vi "HH_ToImageOffline.vi"(0 "Data In":u32[](array[numeric]), 1 "Reset":bool, 2 "Image Array In":i32[][](array[numeric]), 5 "Data Count":i32, 9 "Pixel Time (Laser Pulses)":i32, 11 "Trace Bins":i32=25) -> (3 "Image Array Out":i32[][](array[numeric]), 4 "Histograms":i32[][](array[numeric]), 6 "Total Photon Count":u64[](array[numeric]), 8 "Trigger Times":u64[](array[numeric]), 13 "Total Oveflow Count":u64, 14 "Num Records Total":i64, 15 "Traces":i32[][](array[numeric]))   [LabVIEW 2011]
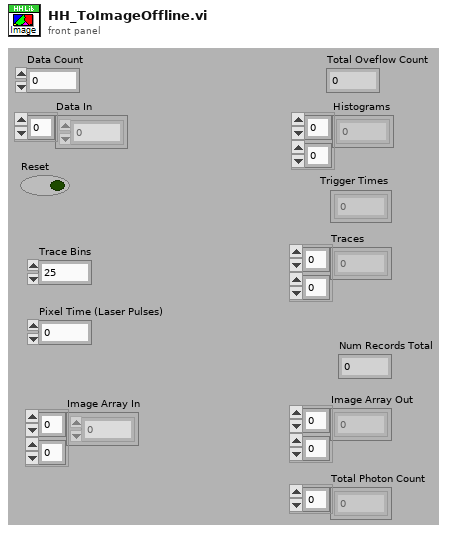
[diagram p1: front panel]
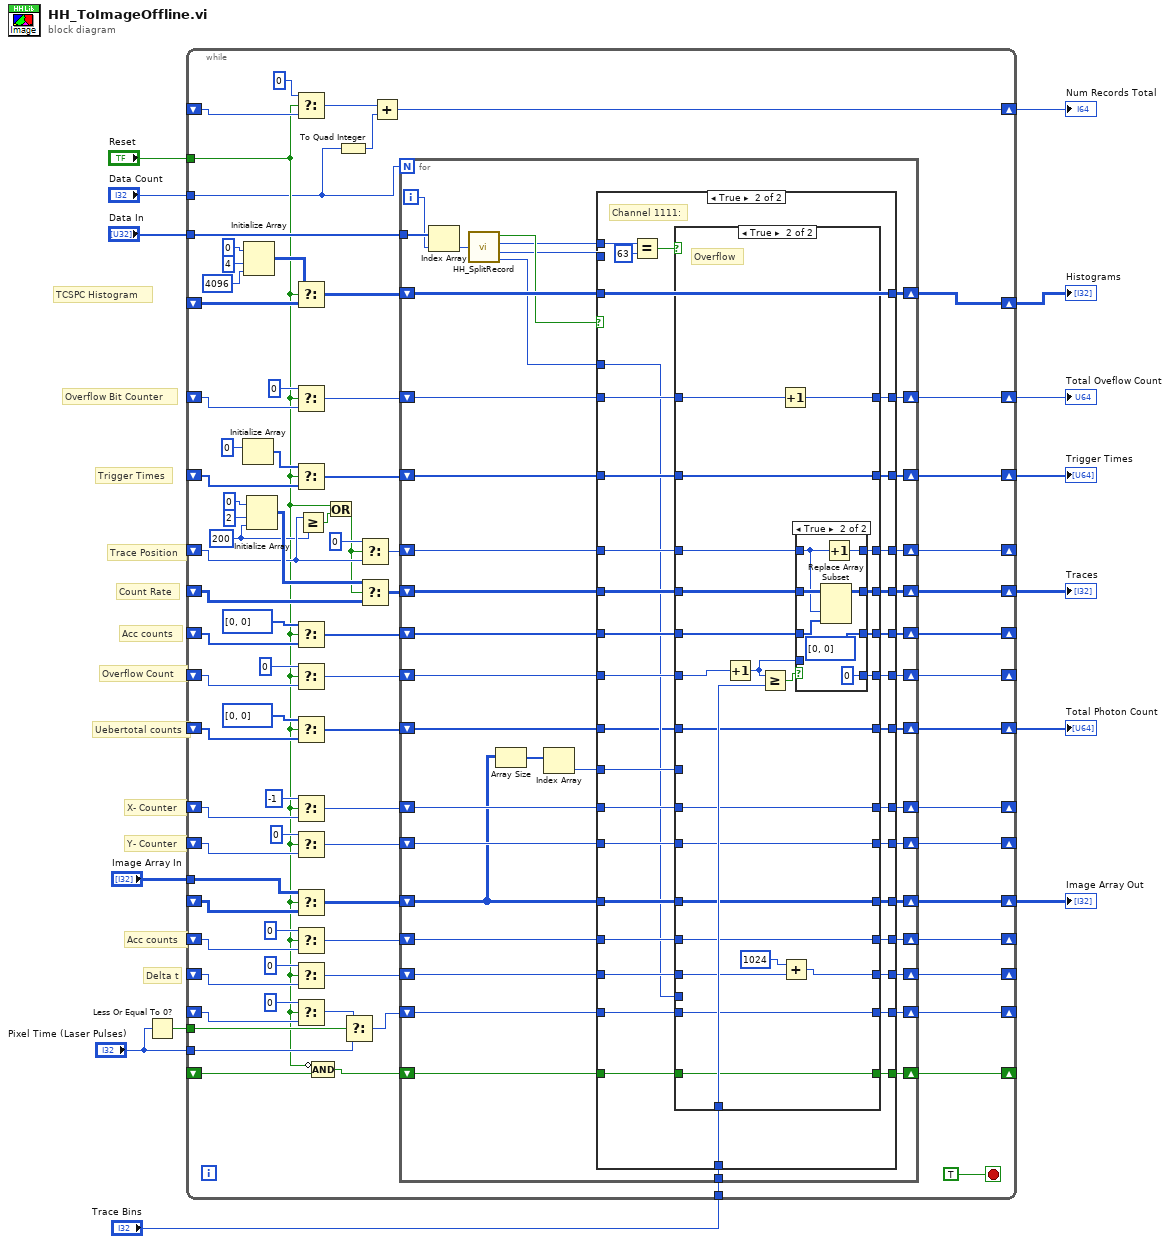
[diagram p0: block diagram]
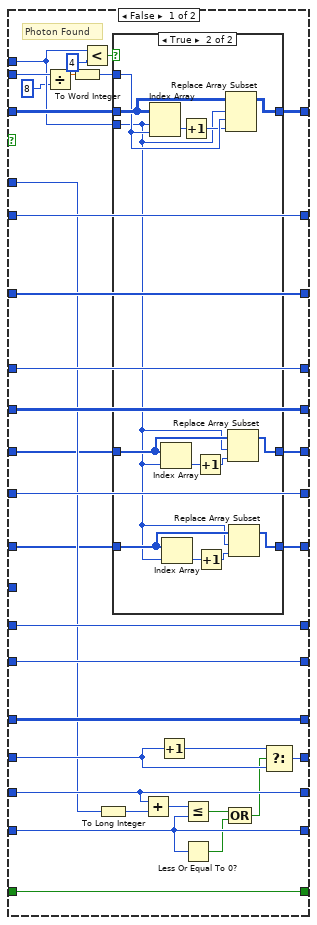
[diagram p2: hidden frame]
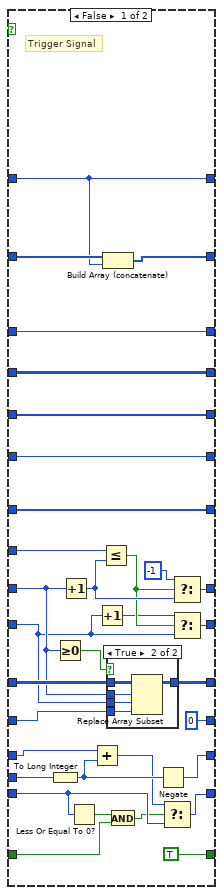
[diagram p4: hidden frame]
diagram:
  # "Uebertotal counts"
  # "Y- Counter"
  # "X- Counter"
  # "Delta t"
  # "Acc counts"
  # "Trace Position"
  # "Overflow Count"
  # "Acc counts"
  # "Count Rate"
  # "Trigger Times"
  # "TCSPC Histogram"
  # "Overflow Bit Counter"
  n1 = Less Or Equal To 0?(x="Pixel Time (Laser Pulses)") -> (x <= 0?=w2:bool)
  n2 = while {
    tunnel: "Data In" -> [w93]
    shift-right: [w94] -> w14
    shift-left: _ -> [w89]
    tunnel: "Reset" -> [w17]
    shift-right: [w86] -> w4
    shift-left: _ -> [w85]
    shift-right: [w81] -> w11
    shift-left: _ -> [w80]
    shift-right: [w76] -> w9
    shift-left: _ -> [w75]
    shift-right: [w73] -> _
    shift-left: _ -> [w72]
    shift-right: [w70] -> _
    shift-left: _ -> [w69]
    tunnel: "Trace Bins" -> [w68]
    shift-right: [w65] -> _
    shift-left: _ -> [w63]
    shift-right: [w59] -> w7
    shift-left: _ -> [w58]
    tunnel: "Image Array In" -> [w61]
    shift-right: [w54] -> _
    shift-left: _ -> [w52]
    shift-right: [w53] -> _
    shift-left: _ -> [w51]
    shift-right: [w46] -> _
    shift-left: _ -> [w44]
    shift-right: [w45] -> _
    shift-left: _ -> [w43]
    tunnel: "Data Count" -> [w16]
    shift-right: [w38] -> w5
    shift-left: _ -> [w40]
    shift-right: [w29] -> w3
    shift-left: _ -> [w28]
    shift-right: [w24] -> _
    shift-left: _ -> [w21]
    tunnel: w2 -> [w26]
    tunnel: "Pixel Time (Laser Pulses)" -> [w25]
    shift-right: [w20] -> _
    shift-left: _ -> [w19]
    stop <- TRUE stop-if-true
    w35 = 200 ("dimension size")
    n3 = Initialize Array(u64 0 ("element")) -> (w83:u64[])  [unwired: 1 out]
    n4 = Initialize Array(0 ("element"), 4 ("dimension size"), 4096 ("dimension size")) -> (w90:i32[][])
    n5 = Initialize Array(0 ("element"), 2 ("dimension size"), w35) -> (w78:i32[][])
    n6 = Select(t=i64 0 ("Data Count 2"), s=w17, f=w40) -> (s? t:f=w39:i64)
    n7 = Select(t=w90, s=w17, f=w89) -> (s? t:f=w91:i32[][])
    n8 = Select(t=u64 0, s=w17, f=w85) -> (s? t:f=w87:u64)
    n9 = Select(t=w83, s=w17, f=w80) -> (s? t:f=w82:u64[])
    n10 = Select(t=u32[] [0, 0] ("initialized array"), s=w17, f=w72) -> (s? t:f=w74:u32[])
    n11 = Select(t=u32 0, s=w17, f=w69) -> (s? t:f=w71:u32)
    n12 = Select(t=u64[] [0, 0] ("initialized array"), s=w17, f=w28) -> (s? t:f=w30:u64[])
    n13 = Select(t=-1, s=w17, f=w44) -> (s? t:f=w48:i32)
    n14 = Select(t=0, s=w17, f=w43) -> (s? t:f=w47:i32)
    n15 = Select(t=w61, s=w17, f=w58) -> (s? t:f=w60:i32[][])
    n16 = Select(t=0, s=w17, f=w52) -> (s? t:f=w56:i32)
    n17 = Select(t=0, s=w17, f=w51) -> (s? t:f=w55:i32)
    n18 = Select(t=0, s=w17, f=w21) -> (s? t:f=w23:i32)
    n19 = Greater Or Equal?(x=w63, y=w35) -> (x >= y?=w64:bool)
    n20 = Compound Arithmetic op=AND(invert w17, w19) -> (w18:bool)
    n21 = Or(x=w17, y=w64) -> (x .or. y?=w62:bool)
    n22 = To Quad Integer(1:w16) -> (0:w15:i64)
    n23 = Select(t=w23, s=w26, f=w25) -> (s? t:f=w27:i32)
    n24 = Select(t=0, s=w62, f=w63) -> (s? t:f=w66:i32)
    n25 = Select(t=w78, s=w62, f=w75) -> (s? t:f=w77:i32[][])
    n26 = Add(x=w39, y=w15) -> (x+y=w38:i64)
    n27 = for {
      N: w16 -> [_]
      tunnel: w93 -> [w107]
      shift-right: [w134] -> w94
      shift-left: w91 -> [w135]
      shift-right: [w132] -> w86
      shift-left: w87 -> [w133]
      shift-right: [w130] -> w81
      shift-left: w82 -> [w131]
      shift-right: [w126] -> w76
      shift-left: w77 -> [w127]
      shift-right: [w128] -> w73
      shift-left: w74 -> [w129]
      shift-right: [w124] -> w70
      shift-left: w71 -> [w125]
      tunnel: w68 -> [w123]
      shift-right: [w121] -> w65
      shift-left: w66 -> [w122]
      shift-right: [w120] -> w59
      shift-left: w60 -> [w112]
      shift-right: [w118] -> w54
      shift-left: w56 -> [w119]
      shift-right: [w116] -> w53
      shift-left: w55 -> [w117]
      shift-right: [w113] -> w46
      shift-left: w48 -> [w114]
      shift-right: [w109] -> w45
      shift-left: w47 -> [w115]
      shift-right: [w104] -> w29
      shift-left: w30 -> [w105]
      shift-right: [w103] -> w24
      shift-left: w27 -> [w108]
      shift-right: [w102] -> w20
      shift-left: w18 -> [w101]
      i -> [w106]
      n28 = Index Array(array=w107, index=w106) -> (element=w100:u32)
      n29 = call "HH_SplitRecord.vi"("Record in"=w100) -> ("Special"=w99:bool, "channel"=w98:i32, "time"=w96:i32, "nsync"=w97:u16)
      n30 = Array Size(array=w112) -> (size(s)=w111:i32[])
      n31 = Index Array(array=w111) -> (element=w110:i32)  [unwired: 1 in]
      n32 = case shown="True" w99 {
        tunnel: w135 -> [w168 w218]
        tunnel: w98 -> [w139 w187]
        tunnel: [w167 w218] -> w134
        tunnel: w96 -> [w140 _]
        tunnel: w133 -> [w166 w220]
        tunnel: [w166 w219] -> w132
        tunnel: w131 -> [w165 w217]
        tunnel: [w165 w216] -> w130
        tunnel: w129 -> [w151 w214]
        tunnel: [w150 w210] -> w128
        tunnel: w127 -> [w164 w213]
        tunnel: [w164 w209] -> w126
        tunnel: w125 -> [w163 w215]
        tunnel: [w163 w211] -> w124
        tunnel: w123 -> [_ w212]
        tunnel: w122 -> [w162 w208]
        tunnel: [w162 w207] -> w121
        tunnel: w112 -> [w161 w205]
        tunnel: [w161 w206] -> w120
        tunnel: w119 -> [w160 w201]
        tunnel: [w159 w202] -> w118
        tunnel: w117 -> [w158 w204]
        tunnel: [w158 w203] -> w116
        tunnel: w115 -> [w157 w200]
        tunnel: w114 -> [w156 w199]
        tunnel: [w156 w198] -> w113
        tunnel: w110 -> [_ w197]
        tunnel: [w157 w196] -> w109
        tunnel: w108 -> [w145 w192]
        tunnel: w97 -> [w153 w195]
        tunnel: w105 -> [w147 w194]
        tunnel: [w146 w193] -> w104
        tunnel: [w145 w191] -> w103
        tunnel: [w141 w190] -> w102
        tunnel: w101 -> [w141 w189]
        frame False {
          # "Photon Found"
          n33 = Divide(x=w140, y=8) -> (x/y=w138:dbl)
          n34 = To Word Integer(number=w138) -> (16bit integer=w136:i16)
          n35 = Less?(x=w139, y=4) -> (x < y?=w149:bool)
          n36 = To Long Integer(number=w153) -> (32bit integer=w152:i32)
          n37 = case shown="True" w149 {
            tunnel: w168 -> [w171 w185]
            tunnel: [w171 w184] -> w167
            tunnel: w136 -> [_ w183]
            tunnel: w139 -> [_ w172]
            tunnel: w151 -> [w170 w182]
            tunnel: [w170 w181] -> w150
            tunnel: w147 -> [w169 w174]
            tunnel: [w169 w173] -> w146
            frame False {
            }
            frame True {
              n38 = Index Array(array=w185, index (row)=w172, index (col)=w183) -> (element=w180:i32)
              n39 = Index Array(array=w182, index=w172) -> (element=w178:u32)
              n40 = Index Array(array=w174, index=w172) -> (element=w176:u64)
              n41 = Increment(x=w180) -> (x+1=w179:i32)
              n42 = Increment(x=w178) -> (x+1=w177:u32)
              n43 = Increment(x=w176) -> (x+1=w175:u64)
              n44 = Replace Array Subset(array=w185, new element=w179, index (row)=w172, index (col)=w183) -> (w184:i32[][])
              n45 = Replace Array Subset(array=w182, new element=w177, index=w172) -> (w181:u32[])
              n46 = Replace Array Subset(array=w174, new element=w175, index=w172) -> (w173:u64[])
            }
          }
          n47 = Add(x=w158, y=w152) -> (x+y=w154:i32)
          n48 = Increment(x=w160) -> (x+1=w155:i32)
          n49 = Less Or Equal?(x=w154, y=w145) -> (x <= y?=w144:bool)
          n50 = Less Or Equal To 0?(x=w145) -> (x <= 0?=w143:bool)
          n51 = Compound Arithmetic op=OR(w144, w143) -> (w142:bool)
          n52 = Select(t=w155, s=w142, f=w160) -> (s? t:f=w159:i32)
        }
        frame True {
          # "Channel 1111:"
          n53 = Equal?(x=w187, y=63) -> (x = y?=w186:bool)
          n54 = case shown="True" w186 {
            tunnel: w220 -> [w251 w282]
            tunnel: [w251 w281] -> w219
            tunnel: w217 -> [w253 w283]
            tunnel: [w252 w283] -> w216
            tunnel: w215 -> [w250 w266]
            tunnel: w214 -> [w249 w277]
            tunnel: w213 -> [w248 w275]
            tunnel: w212 -> [_ w280]
            tunnel: [w250 w278] -> w211
            tunnel: [w249 w276] -> w210
            tunnel: [w248 w274] -> w209
            tunnel: w208 -> [w247 w273]
            tunnel: [w247 w272] -> w207
            tunnel: [w245 w271] -> w206
            tunnel: w205 -> [w246 w271]
            tunnel: w204 -> [w230 w264]
            tunnel: [w232 w260] -> w203
            tunnel: [0 ("t") w269] -> w202
            tunnel: w201 -> [w244 w269]
            tunnel: w195 -> [w229 _]
            tunnel: w200 -> [w234 w268]
            tunnel: w199 -> [w239 w267]
            tunnel: [w241 w267] -> w198
            tunnel: w197 -> [w240 _]
            tunnel: [w235 w268] -> w196
            tunnel: w194 -> [w231 w263]
            tunnel: [w231 w263] -> w193
            tunnel: w192 -> [w226 w262]
            tunnel: [w225 w262] -> w191
            tunnel: [TRUE w261] -> w190
            tunnel: w189 -> [w221 w261]
            frame False {
              # "Trigger Signal"
              n55 = To Long Integer(number=w229) -> (32bit integer=w228:i32)
              n56 = Greater Or Equal To 0?(x=w239) -> (x >= 0?=w242:bool)
              n57 = Increment(x=w239) -> (x+1=w238:i32)
              n58 = Less Or Equal To 0?(x=w226) -> (x <= 0?=w224:bool)
              n59 = Add(x=w230, y=w228) -> (x+y=w227:i32)
              n60 = Increment(x=w234) -> (x+1=w233:i32)
              n61 = Less Or Equal?(x=w240, y=w238) -> (x <= y?=w236:bool)
              n62 = Build Array (concatenate)(w253, w251) -> (w252:u64[])
              n63 = case shown="True" w242 {
                tunnel: w246 -> [w254 w259]
                tunnel: [w254 w258] -> w245
                tunnel: w244 -> [_ w257]
                tunnel: w234 -> [_ w256]
                tunnel: w239 -> [_ w255]
                frame False {
                }
                frame True {
                  n64 = Replace Array Subset(array=w259, new element=w257, index (row)=w255, index (col)=w256) -> (w258:i32[][])
                }
              }
              n65 = And(x=w224, y=w221) -> (x .and. y?=w223:bool)
              n66 = Negate(x=w228) -> (-x=w232:i32)
              n67 = Select(t=w227, s=w223, f=w226) -> (s? t:f=w225:i32)
              n68 = Select(t=-1, s=w236, f=w238) -> (s? t:f=w241:i32)
              n69 = Select(t=w233, s=w236, f=w234) -> (s? t:f=w235:i32)
            }
            frame True {
              # "Overflow"
              n70 = Increment(x=w266) -> (x+1=w265:u32)
              n71 = Greater Or Equal?(x=w265, y=w280) -> (x >= y?=w279:bool)
              n72 = Increment(x=w282) -> (x+1=w281:u64)
              n73 = Add(x=1024 ("t"), y=w264) -> (x+y=w260:i32)
              n74 = case shown="True" w279 {
                tunnel: w265 -> [w287 _]
                tunnel: [w287 u32 0] -> w278
                tunnel: w277 -> [w286 w292]
                tunnel: [w286 u32[] [0, 0] ("initialized array")] -> w276
                tunnel: w275 -> [w285 w293]
                tunnel: [w285 w291] -> w274
                tunnel: w273 -> [w284 w289]
                tunnel: [w284 w290] -> w272
                frame False {
                }
                frame True {
                  n75 = Replace Array Subset(array=w293, new element=w292, index (col)=w289) -> (w291:i32[][])  [unwired: 1 in]
                  n76 = Increment(x=w289) -> (x+1=w290:i32)
                }
              }
            }
          }
        }
      }
    }
  }
  "Histograms" <- w14
  "Trigger Times" <- w11
  "Traces" <- w9
  "Image Array Out" <- w7
  "Num Records Total" <- w5
  "Total Oveflow Count" <- w4
  "Total Photon Count" <- w3
